vi "Get Plot Visibility (WFGraph).vi"(8 "error in (no error)":errorcluster, 10 "ActPlot":i32, 11 "WFGraph in":refnum<vi>) -> (0 "error out":errorcluster, 1 "Plot.Visible?":bool, 2 "Active Plot":i32)   [LabVIEW 2019, in "Instrument UI.Lockin.lvclass"]
uses:
  Instrument UI.Lockin.lvclass
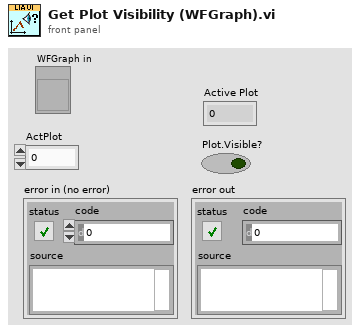
[diagram p1: front panel]
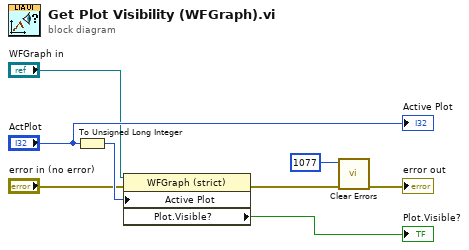
[diagram p0: block diagram]
diagram:
  n1 = To Unsigned Long Integer(number="ActPlot") -> (unsigned 32bit integer=w4:u32)
  n2 = property on="Property Node" class="WFGraph (strict)"(reference="WFGraph in", error in="error in (no error)", "Active Plot"=w4) -> (error out=w2:errorcluster, "Plot.Visible?"=→"Plot.Visible?":bool)  [unwired: 1 out]
  n3 = call <vilib>:"Clear Errors.vi"("error in (no error)"=w2, "specific error code to clear (0: all)"=1077) -> ("error out"=→"error out":errorcluster)  [unwired: 4 in, 1 out]
  "Active Plot" <- "ActPlot"
